vi "AutofocusOptions_wip.vi"() -> ()   [LabVIEW 2019]
uses:
  <vilib>/userDefined/High Color/IMAQdx.ctl
  <vilib>/Utility/file.llb/Read Delimited Spreadsheet (DBL).vi
  <vilib>/vision/driver/NI_Vision_Acquisition_Software.lvlib
panel:
  in  "Camera":T1="cam1"
  in  "DistSensorInTextFileMode":bool
  out "XYZ_NiterOrDistSenErr":string
  in  "AbortAutoFocus":bool
  in  "Tolerance":dbl=0.005 format="%#_13g"
  out "TimeTaken":dbl
  out "Z":string
  in  "SafeMaxZ":dbl=75.0 format="%#_13g"
  out "N_iterations":dbl[](array[numeric])
  in  "InitialStepSize":dbl=0.1
  out "HighVSPosition":picture
  in  "Z OutputFile":path=path "C:/Users/TTUHEP/Documents/LabVIEW/GantryPrograms/LogFiles/temp.txt"
  in  "PlotOutputFile":string="C:\\Users\\TTUHEP\\Documents\\LabVIEW\\GantryPrograms\\LogFiles\\plot.png"
  in  "Zoffset_textFile":dbl
  out "Image":T2(plugin-control)
  in  "InitialPositions":path=path "C:/Users/TTUHEP/Documents/LabVIEW/GantryPrograms/Configs/A1_BP_HeightMeasure.txt"
  out "error out":errorcluster
  out "BestZvalue":dbl
  in  "error in (no error)":errorcluster
  in  "Z":dbl=68.683
  in  "Y":dbl=1011.604463
  in  "X":dbl=288.7508563
  in  "ControlType":T3(ring)=enum."SinglePoint" caption="Operation Mode"
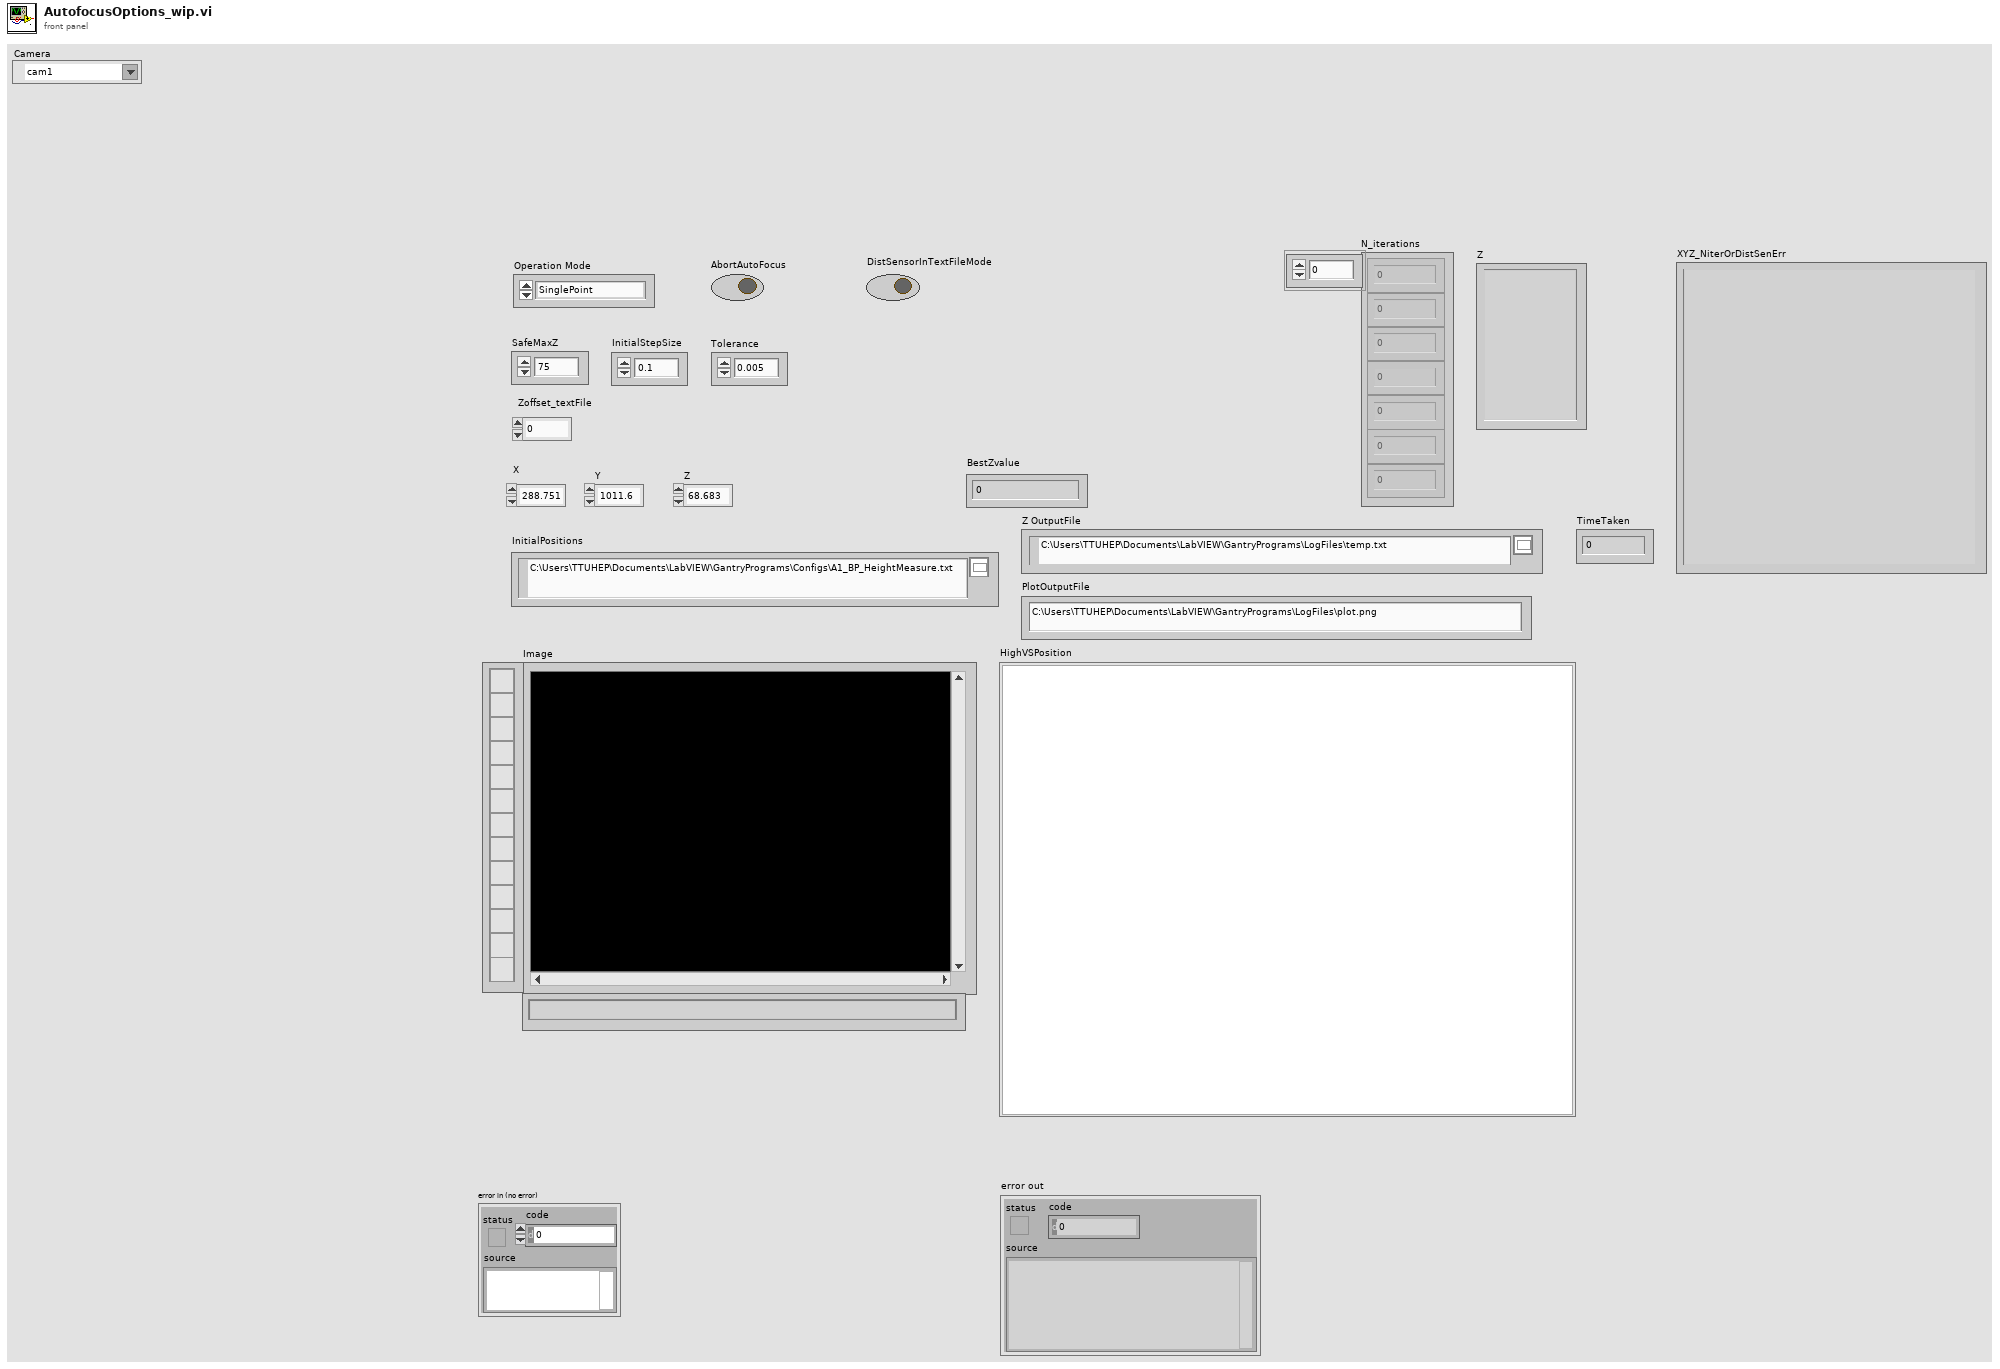
[diagram p1: front panel]
types:
  T1 = typedef "IMAQdx.ctl" = refnum<k21>
  T2 = typedef "IMAQ Image.ctl" = refnum<image>
  T3 = enum16{"CurrentPosition", "SinglePoint", "TextFile"}
  T4 = typedef "Image Type" = u32
  T5 = enum16{"open", "replace", "create", "open or create", "replace or create", "replace or create with confirmation"}
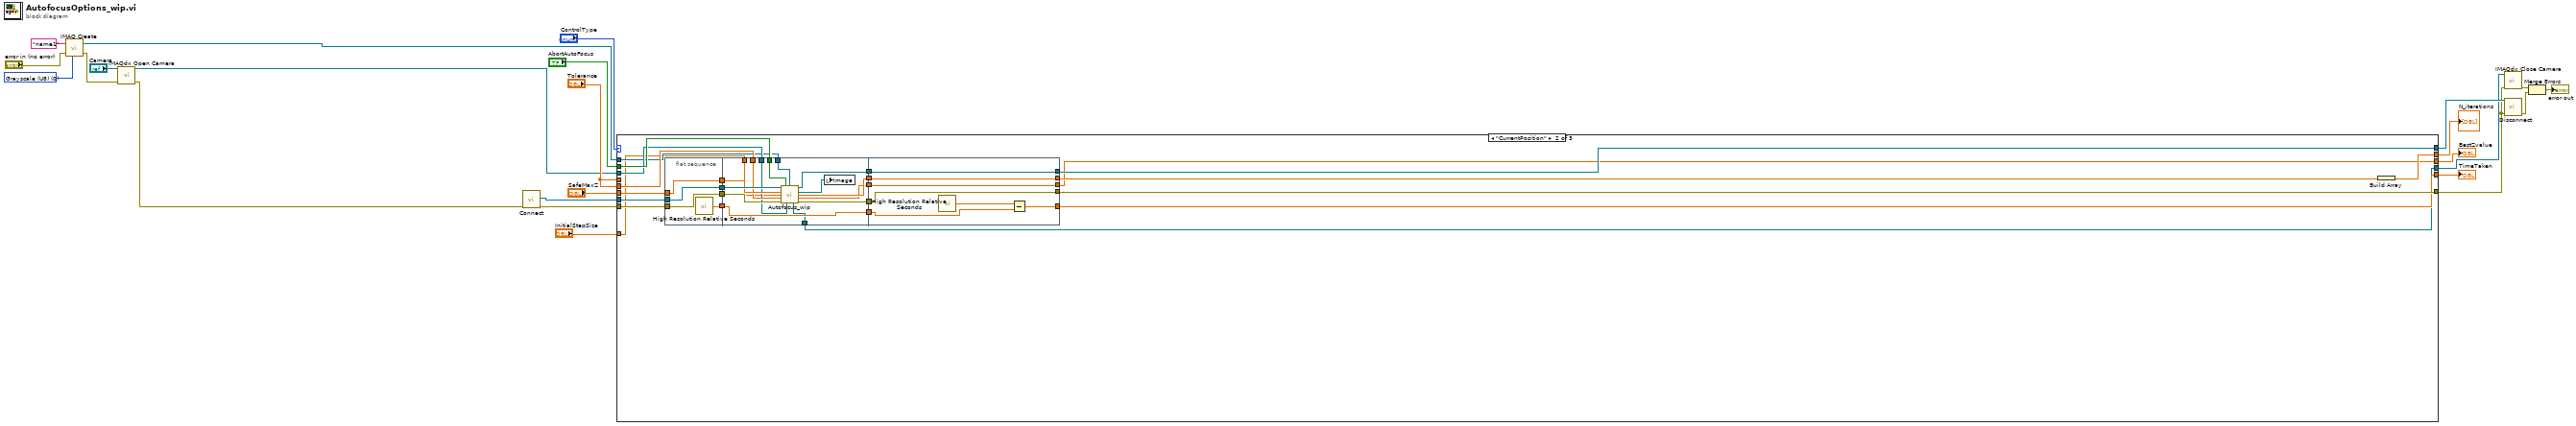
[diagram p0: block diagram]
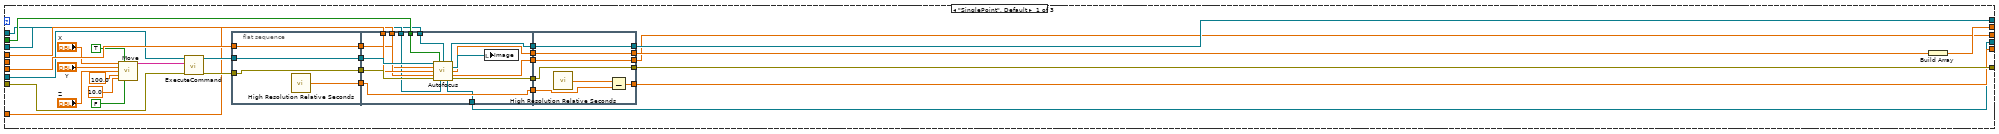
[diagram p2: hidden frame]
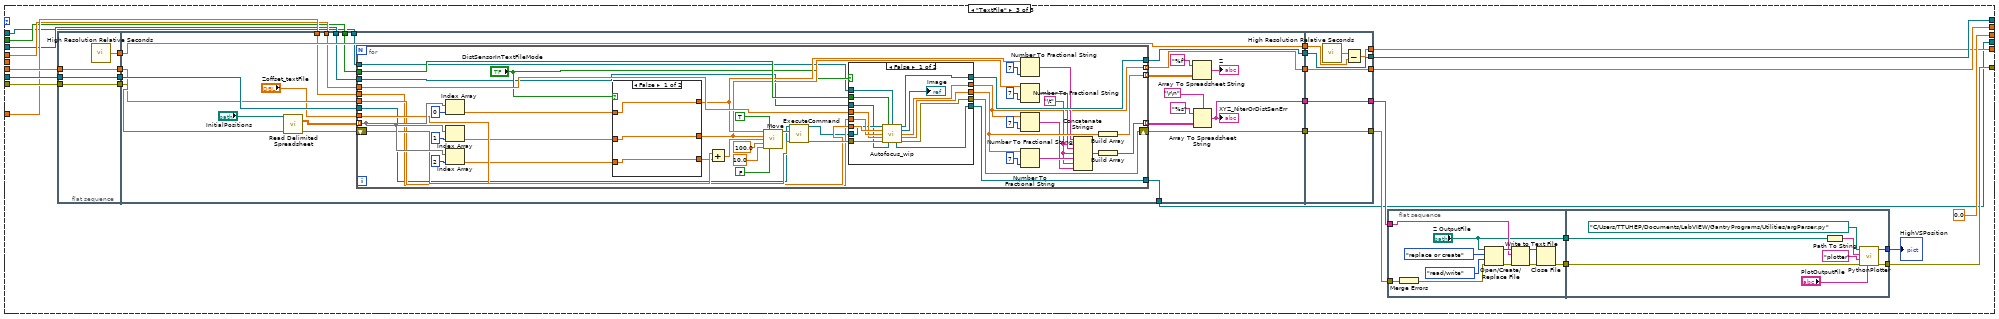
[diagram p3: hidden frame]
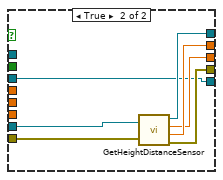
[diagram p4: hidden frame]
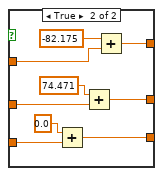
[diagram p5: hidden frame]
diagram:
  w10 = T4 0 items=["Grayscale (U8)", "Grayscale (I16)", "Grayscale (SGL)", "Complex (CSG)", "RGB (U32)", "HSL (U32)", "RGB (U64)", "Grayscale (U16)"] ("Image Type")
  n1 = call "IMAQ Create"("Image Name"="name1" ("ImageName"), "Image Type"=w10, "error in (no error)"="error in (no error)") -> ("New Image"=w3:T2, "error out"=w12:errorcluster)  [unwired: 2 in]
  n2 = call <vilib>:"IMAQdx Open Camera.vi"("error in"=w12, "Session In"="Camera") -> ("error out"=w1:errorcluster, "Session Out"=w2:T1)  [unwired: 8 in]
  n3 = call "Connect.vi"("error in (no error)"=w1) -> ("error out"=w22:errorcluster, "controller"=w23:refnum<k24>)  [unwired: 9 in]
  n4 = case shown="\"CurrentPosition\"" "ControlType" {
    tunnel: w22 -> [w32 w106 w157]
    tunnel: [w58 w102 w153] -> w6
    tunnel: w23 -> [w42 w107 w161]
    tunnel: [w57 w103 w160] -> w21
    tunnel: [w55 w104 w158] -> w20
    tunnel: "SafeMaxZ" -> [w54 w105 w156]
    tunnel: [w53 w101 0.0 ("BestZvalue")] -> w18
    tunnel: [w43 w91 w141] -> w17
    tunnel: "Tolerance" -> [_ w90 _]
    tunnel: "InitialStepSize" -> [w30 w85 w140]
    tunnel: "Tolerance" -> [w29 _ w139]
    tunnel: "AbortAutoFocus" -> [w28 w89 w138]
    tunnel: w2 -> [w27 w88 w137]
    tunnel: w3 -> [w26 w87 w136]
    tunnel: [w25 w86 w135] -> w8
    frame "SinglePoint", Default {
      n5 = call "Move.vi"("X"="X", "Absolute"=TRUE, "Y"="Y", "Z"="Z", "SpeedXY (mm/s)"=100.0, "SpeedZ (mm/s)"=10.0, "Move Z first"=FALSE) -> ("Position Gcode"=w33:string)  [unwired: 8 in]
      n6 = call "ExecuteCommand.vi"("error in (no error)"=w32, "Command Code"=w33, "controller in"=w42) -> ("error out"=w31:errorcluster, "controller out"=w41:refnum<k24>)  [unwired: 6 in, 1 out]
      n7 = flat-sequence {
        tunnel: w54 -> [w61]
        tunnel: w41 -> [w62]
        tunnel: [w59] -> w52
        tunnel: [w62] -> w51
        tunnel: [w61] -> w50
        tunnel: [w60] -> w44
        tunnel: w31 -> [w59]
        tunnel: w52 -> [w77]
        tunnel: w51 -> [w70]
        tunnel: w50 -> [w67]
        tunnel: [w76] -> w49
        tunnel: [w75] -> w48
        tunnel: [w73] -> w47
        tunnel: [w72] -> w46
        tunnel: [w71] -> w45
        tunnel: w44 -> [w71]
        tunnel: w30 -> [w69]
        tunnel: w29 -> [w68]
        tunnel: w28 -> [w66]
        tunnel: w27 -> [w65]
        tunnel: w26 -> [w64]
        tunnel: [w63] -> w25
        tunnel: [w81] -> w53
        tunnel: [w82] -> w56
        tunnel: [w83] -> w57
        tunnel: [w84] -> w58
        tunnel: w49 -> [w84]
        tunnel: w48 -> [w83]
        tunnel: w47 -> [w82]
        tunnel: w46 -> [w81]
        tunnel: w45 -> [w79]
        tunnel: [w78] -> w43
        frame #0 {
          n8 = call <vilib>:"High Resolution Relative Seconds.vi"() -> ("relative seconds"=w60:dbl)
        }
        frame #1 {
          n9 = call "Autofocus.vi"("controller in"=w70, "AbortAutoFocus"=w66, "ImageIn"=w64, "SafeMaxZ"=w67, "InitialStepSize"=w69, "Tolerance"=w68, "error in (no error)"=w77, "SessionIn"=w65) -> ("controller out"=w75:refnum<k24>, "Image"=w74:T2, "N_iterations"=w73:dbl, "BestZvalue"=w72:dbl, "Session Out"=w63:T1, "error out"=w76:errorcluster)  [unwired: 2 in]
          n10 = local write "Image"(w74) -> ()
        }
        frame #2 {
          n11 = call <vilib>:"High Resolution Relative Seconds.vi"() -> ("relative seconds"=w80:dbl)
          n12 = Subtract(x=w80, y=w79) -> (x-y=w78:dbl)
        }
      }
      n13 = Build Array(w56) -> (w55:dbl[])
    }
    frame "CurrentPosition" {
      n14 = flat-sequence {
        tunnel: w105 -> [w110]
        tunnel: w106 -> [w111]
        tunnel: w107 -> [w112]
        tunnel: [w112] -> w100
        tunnel: [w111] -> w99
        tunnel: [w110] -> w98
        tunnel: [w109] -> w93
        tunnel: w100 -> [w121]
        tunnel: w99 -> [w120]
        tunnel: w98 -> [w119]
        tunnel: [w126] -> w97
        tunnel: [w125] -> w96
        tunnel: [w124] -> w95
        tunnel: [w123] -> w94
        tunnel: w93 -> [w122]
        tunnel: [w122] -> w92
        tunnel: w90 -> [w118]
        tunnel: w89 -> [w117]
        tunnel: w88 -> [w116]
        tunnel: w87 -> [w115]
        tunnel: [w114] -> w86
        tunnel: w85 -> [w113]
        tunnel: [w131] -> w101
        tunnel: [w132] -> w102
        tunnel: [w133] -> w103
        tunnel: [w134] -> w108
        tunnel: w97 -> [w134]
        tunnel: w96 -> [w133]
        tunnel: w95 -> [w132]
        tunnel: w94 -> [w131]
        tunnel: w92 -> [w129]
        tunnel: [w128] -> w91
        frame #0 {
          n15 = call <vilib>:"High Resolution Relative Seconds.vi"() -> ("relative seconds"=w109:dbl)
        }
        frame #1 {
          n16 = call "Autofocus_wip.vi"("controller in"=w121, "AbortAutoFocus"=w117, "ImageIn"=w115, "SafeMaxZ"=w119, "InitialStepSize"=w113, "Tolerance"=w118, "error in (no error)"=w120, "SessionIn"=w116) -> ("controller out"=w125:refnum<k24>, "Image"=w127:T2, "N_iterations"=w126:dbl, "BestZvalue"=w123:dbl, "Session Out"=w114:T1, "error out"=w124:errorcluster)  [unwired: 2 in]
          n17 = local write "Image"(w127) -> ()
        }
        frame #2 {
          n18 = call <vilib>:"High Resolution Relative Seconds.vi"() -> ("relative seconds"=w130:dbl)
          n19 = Subtract(x=w130, y=w129) -> (x-y=w128:dbl)
        }
      }
      n20 = Build Array(w108) -> (w104:dbl[])
    }
    frame "TextFile" {
      n21 = flat-sequence {
        tunnel: w156 -> [w164]
        tunnel: w157 -> [w165]
        tunnel: w161 -> [w166]
        tunnel: [w166] -> w150
        tunnel: [w165] -> w149
        tunnel: [w164] -> w148
        tunnel: [w163] -> w143
        tunnel: w150 -> [w188]
        tunnel: w149 -> [w184]
        tunnel: w148 -> [w182]
        tunnel: [w171] -> w147
        tunnel: [w187] -> w146
        tunnel: [w167] -> w145
        tunnel: [w185] -> w144
        tunnel: w143 -> [w179]
        tunnel: [w179] -> w142
        tunnel: w140 -> [w178]
        tunnel: w139 -> [w177]
        tunnel: w138 -> [w176]
        tunnel: w137 -> [w170]
        tunnel: w136 -> [w169]
        tunnel: [w168] -> w135
        tunnel: [w272] -> w158
        tunnel: [w273] -> w159
        tunnel: [w274] -> w160
        tunnel: [w275] -> w162
        tunnel: w147 -> [w275]
        tunnel: w146 -> [w274]
        tunnel: w145 -> [w273]
        tunnel: w144 -> [w272]
        tunnel: w142 -> [w270]
        tunnel: [w269] -> w141
        frame #0 {
          n22 = call <vilib>:"High Resolution Relative Seconds.vi"() -> ("relative seconds"=w163:dbl)
        }
        frame #1 {
          n23 = call-poly <vilib>:"Read Delimited Spreadsheet.vi"("file path (dialog if empty)"="InitialPositions", "error in (no error)"=w184) -> ("all rows"=w190:dbl[][], "error out"=w183:errorcluster)  [unwired: 8 in, 4 out]
          n24 = for {
            tunnel: w190 -> [w232] mode=indexing
            tunnel: [w231] -> w180 mode=indexing
            tunnel: w188 -> [w217]
            tunnel: [w230] -> w187
            tunnel: [w196] -> w185 mode=indexing
            tunnel: w182 -> [w220]
            tunnel: "Zoffset_textFile" -> [w229]
            tunnel: w178 -> [w219]
            tunnel: w177 -> [w218]
            tunnel: w176 -> [w215]
            tunnel: [w206] -> w175 mode=indexing
            shift-right: [w205] -> w171
            shift-left: w183 -> [w222]
            tunnel: w170 -> [w193]
            tunnel: w169 -> [w192]
            tunnel: [w191] -> w168
            w197 = "\t"
            n25 = Index Array(array=w232, index=0) -> (element=w203:dbl)
            n26 = Index Array(array=w232, index=1) -> (element=w201:dbl)
            n27 = Index Array(array=w232, index=2) -> (element=w200:dbl)
            n28 = case shown="False" "DistSensorInTextFileMode" {
              tunnel: [w259 w267] -> w204
              tunnel: w203 -> [w259 w266]
              tunnel: [w258 w265] -> w202
              tunnel: w201 -> [w258 w263]
              tunnel: w200 -> [w257 w262]
              tunnel: [w257 w260] -> w199
              frame False {
              }
              frame True {
                n29 = Add(x=0.0, y=w262) -> (x+y=w260:dbl)
                n30 = Add(x=74.471, y=w263) -> (x+y=w265:dbl)
                n31 = Add(x=-82.175, y=w266) -> (x+y=w267:dbl)
              }
            }
            n32 = Add(x=w229, y=w199) -> (x+y=w228:dbl)
            n33 = call "Move.vi"("X"=w204, "Absolute"=TRUE, "Y"=w202, "Z"=w228, "SpeedXY (mm/s)"=100.0, "SpeedZ (mm/s)"=10.0, "Move Z first"=FALSE) -> ("Position Gcode"=w223:string)  [unwired: 8 in]
            n34 = call "ExecuteCommand.vi"("error in (no error)"=w222, "Command Code"=w223, "controller in"=w217) -> ("error out"=w221:errorcluster, "controller out"=w216:refnum<k24>)  [unwired: 6 in, 1 out]
            n35 = case shown="False" "DistSensorInTextFileMode" {
              tunnel: [w249 w254] -> w230
              tunnel: [w248 w252] -> w196
              tunnel: w221 -> [w246 w255]
              tunnel: w220 -> [w245 _]
              tunnel: w219 -> [w244 _]
              tunnel: w218 -> [w243 _]
              tunnel: w216 -> [w242 w256]
              tunnel: w215 -> [w241 _]
              tunnel: [w240 w251] -> w212
              tunnel: [w239 w253] -> w205
              tunnel: w193 -> [w238 w250]
              tunnel: w192 -> [w237 _]
              tunnel: [w236 w250] -> w191
              frame False {
                n36 = call "Autofocus_wip.vi"("controller in"=w242, "AbortAutoFocus"=w241, "ImageIn"=w237, "SafeMaxZ"=w245, "InitialStepSize"=w244, "Tolerance"=w243, "error in (no error)"=w246, "SessionIn"=w238) -> ("controller out"=w249:refnum<k24>, "Image"=→"Image":T2, "N_iterations"=w248:dbl, "BestZvalue"=w240:dbl, "Session Out"=w236:T1, "error out"=w239:errorcluster)  [unwired: 2 in]
              }
              frame True {
                n37 = call "GetHeightDistanceSensor.vi"("controller in"=w256, "error in (no error)"=w255) -> ("controller out"=w254:refnum<k24>, "MeanHeight(mm)"=w251:dbl, "SDofHeight(mm)"=w252:dbl, "error out"=w253:errorcluster)
              }
            }
            n38 = Number To Fractional String(number=w204, precision (6)=i16 7) -> (F-format string=w210:string)  [unwired: 2 in]
            n39 = Number To Fractional String(number=w202, precision (6)=i16 7) -> (F-format string=w209:string)  [unwired: 2 in]
            n40 = Number To Fractional String(number=w196, precision (6)=i16 7) -> (F-format string=w194:string)  [unwired: 2 in]
            n41 = Number To Fractional String(number=w212, precision (6)=i16 7) -> (F-format string=w208:string)  [unwired: 2 in]
            n42 = Concatenate Strings(w210, w197, w209, w197, w208, w197, w194) -> (w207:string)
            n43 = Build Array(w212) -> (w231:dbl[])
            n44 = Build Array(w207) -> (w206:string[])
          }
          n45 = Array To Spreadsheet String(array=w180, 3:"%f" ("format string")) -> (spreadsheet string=→"Z":string)  [unwired: 1 in]
          n46 = Array To Spreadsheet String(delimiter (Tab)="\r\n", array=w175, 3:"%s" ("format string")) -> (spreadsheet string=w167:string)
          "XYZ_NiterOrDistSenErr" <- w167
        }
        frame #2 {
          n47 = call <vilib>:"High Resolution Relative Seconds.vi"() -> ("relative seconds"=w271:dbl)
          n48 = Subtract(x=w271, y=w270) -> (x-y=w269:dbl)
        }
      }
      n49 = flat-sequence {
        tunnel: w162 -> [w286]
        tunnel: w159 -> [w279]
        tunnel: [w277] -> w154
        tunnel: ["Z OutputFile"] -> w151
        tunnel: w154 -> [w294]
        tunnel: [w293] -> w153
        tunnel: [w292] -> w152
        tunnel: w151 -> [w288]
        frame #0 {
          n50 = Merge Errors(w286) -> (w278:errorcluster)
          n51 = Open/Create/Replace File(file path (use dialog)="Z OutputFile", error in=w278, operation (0:open)=T5."replace or create", access (0:read/write)=enum16{"read/write", "read-only", "write-only"}."read/write") -> (refnum out=w282:refnum<file>, error out=w283:errorcluster)  [unwired: 2 in, 1 out]
          n52 = Write to Text File(file (use dialog)=w282, text=w279, error in=w283) -> (refnum out=w285:refnum<file>, error out=w284:errorcluster)  [unwired: 1 in, 1 out]
          n53 = Close File(refnum=w285, error in=w284) -> (error out=w277:errorcluster)  [unwired: 1 out]
        }
        frame #1 {
          n54 = Path To String(path=w288) -> (string=w289:string)
          n55 = call "PythonPlotter.vi"("Output File"="PlotOutputFile", "error in (no error)"=w294, "Function Name"="plotter", "Input File"=w289, "Python Path"=path "C:/Users/TTUHEP/Documents/LabVIEW/GantryPrograms/Utilities/argParser.py") -> ("error out"=w293:errorcluster, "HighVSPosition"=w292:picture)  [unwired: 4 in]
        }
      }
      "HighVSPosition" <- w152
    }
  }
  "N_iterations" <- w20
  "BestZvalue" <- w18
  "TimeTaken" <- w17
  n56 = call <vilib>:"IMAQdx Close Camera.vi"("error in"=w6, "Session In"=w8) -> ("error out"=w7:errorcluster)  [unwired: 9 in]
  n57 = call "Disconnect.vi"("error in (no error)"=w6, "controller"=w21) -> ("error out"=w5:errorcluster)  [unwired: 9 in]
  n58 = Merge Errors(w7, w5) -> (→"error out":errorcluster)
